vi "Topic Prefix.vi"(11 "Topic":string) -> (1 "SN":string, 3 "Topic":string)   [LabVIEW 2018, in "MQTT Messages.lvlib"]
uses:
  MQTT Messages.lvlib
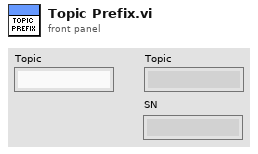
[diagram p1: front panel]
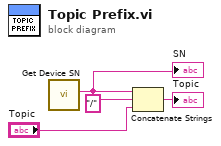
[diagram p0: block diagram]
diagram:
  n1 = call "Get Device SN.vi"() -> ("SN"=w1:string)  [unwired: 10 in, 1 out]
  "SN" <- w1
  n2 = Concatenate Strings(w1, "/" ("string"), "Topic") -> (→"Topic":string)
